vi "Constrained IRF Amplitude Gradient Array.vi"(8 "Error In":errorcluster, 9 "Independent Last Amplitude":bool, 11 "dfai Array":dbl[](array[numeric])) -> (0 "Error Out":errorcluster, 3 "dfai Array":dbl[](array[numeric]))   [LabVIEW 2021, in "Fits.lvlib"]
uses:
  Fits.lvlib
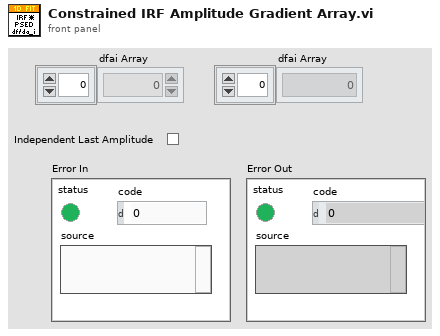
[diagram p1: front panel]
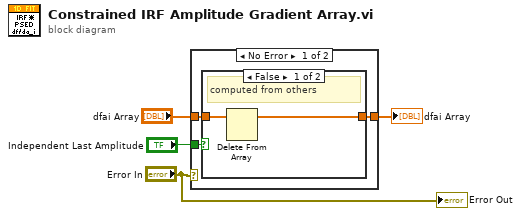
[diagram p0: block diagram]
diagram:
  n1 = case shown="No Error" "Error In" {
    tunnel: [w7 w11] -> w4
    tunnel: "dfai Array" -> [w6 w11]
    tunnel: "Independent Last Amplitude" -> [w5 _]
    frame No Error {
      n2 = case shown="False" w5 {
        tunnel: [w9 w10] -> w7
        tunnel: w6 -> [w8 w10]
        frame False {
          # "computed from others"
          n3 = Delete From Array(array=w8) -> (array with subset deleted=w9:dbl[])  [unwired: 2 in, 1 out]
        }
        frame True {
          # "treated as an indpt param."
        }
      }
    }
    frame Error {
    }
  }
  "dfai Array" <- w4
  "Error Out" <- "Error In"
